vi "Waveform (G3)-Create.vi"(6 "Rep Num":i32, 7 "Name":string, 8 "error in (no error)":errorcluster, 9 "Npts":i32, 10 "Sampling Rate (Hz)":dbl, 11 "Waveform":T1={"Type"=enum."Tone", "Tone"={"Frequency (kHz)"=0.0, "Phase (cycles)"=0.0, "Random phase"=FALSE}, "Pulse Train"={"Pulse width (us)"=0.0, "Pulse rate (Hz)"=0.0, "Gap (ms)"=0.0, "Polarity"=enum."POS", "PT State"={"Template"=[], "Nperiod"=0, "Index"=0, "Pulse Rate (Hz)"=0.0, "Phase (cycles)"=0.0, "Noff"=0}, "Asynch"=FALSE}, "Noise"={"Properties"={"InvFilt"=FALSE, "Aweight"=FALSE, "Seed"=0, "Tokens"=0, "Brickwall"=FALSE}, "Data"={"TokenNum"=0}}, "File"={"Filename"=path "", "Signal"=[], "Channel"=0, "stream"=FALSE, "offset"=0, "nreps"=0, "loops"=0, "Randomize"=FALSE, "order"=[], "Seed"=0, "Tokens"=0}, "FMSweep"={"Rate (oct/s)"=0.0, "Fmin (Hz)"=0.0, "Fmax (Hz)"=0.0, "Ramp (ms)"=0.0, "Linear"=FALSE}, "Chirp Train"={"Params"={"Fmin (kHz)"=4.0, "Fmax (kHz)"=64.0, "Compensate"=FALSE, "Duration (ms)"=2.0}, "Data"={"WF"=[]}}, "Complex Tone"={"Params"={"F0 (Hz)"=0.0, "Band"={"Flow (Hz)"=0.0, "Fhigh (Hz)"=0.0}, "Phase"=enum."Cosine", "Min F0 (Hz)"=0.0, "Max F0 (Hz)"=0.0, "ContinRandPhase"=FALSE, "Max peak factor"=inf, "Max mod depth"=2.0, "MinHarmNum"=0, "MaxHarmNum"=0, "Level Mode"=enum."per component", "% jitter"=0.0}, "Data"={"Ncomp"=0, "MinHarm"=0, "Phase"=[], "Amplitude"=[], "Npts/frame"=0, "Last F0"=0.0, "Fmin"=0.0, "Fmax"=0.0, "Lslope"=0.0, "randphase"=FALSE, "overall rms"=FALSE, "fmult"=[], "jittered"=FALSE}}, "FM"={"Carrier (kHz)"=0.0, "ModRate (Hz)"=0.0, "Depth (Hz)"=0.0, "Phase (cycles)"=0.0}, "Vowel"={"Freqs"="", "Set level"=enum."Total", "Freq"=[], "weights"=[]}, "Ramp"={"Duration (ms)"=0.0}}) -> (0 "error out":errorcluster, 2 "Signal":dbl[](array[numeric]), 3 "Waveform out":T1={"Type"=enum."Tone", "Tone"={"Frequency (kHz)"=0.0, "Phase (cycles)"=0.0, "Random phase"=FALSE}, "Pulse Train"={"Pulse width (us)"=0.0, "Pulse rate (Hz)"=0.0, "Gap (ms)"=0.0, "Polarity"=enum."POS", "PT State"={"Template"=[], "Nperiod"=0, "Index"=0, "Pulse Rate (Hz)"=0.0, "Phase (cycles)"=0.0, "Noff"=0}, "Asynch"=FALSE}, "Noise"={"Properties"={"InvFilt"=FALSE, "Aweight"=FALSE, "Seed"=0, "Tokens"=0, "Brickwall"=FALSE}, "Data"={"TokenNum"=0}}, "File"={"Filename"=path "", "Signal"=[], "Channel"=0, "stream"=FALSE, "offset"=0, "nreps"=0, "loops"=0, "Randomize"=FALSE, "order"=[], "Seed"=0, "Tokens"=0}, "FMSweep"={"Rate (oct/s)"=0.0, "Fmin (Hz)"=0.0, "Fmax (Hz)"=0.0, "Ramp (ms)"=0.0, "Linear"=FALSE}, "Chirp Train"={"Params"={"Fmin (kHz)"=4.0, "Fmax (kHz)"=64.0, "Compensate"=FALSE, "Duration (ms)"=2.0}, "Data"={"WF"=[]}}, "Complex Tone"={"Params"={"F0 (Hz)"=0.0, "Band"={"Flow (Hz)"=0.0, "Fhigh (Hz)"=0.0}, "Phase"=enum."Cosine", "Min F0 (Hz)"=0.0, "Max F0 (Hz)"=0.0, "ContinRandPhase"=FALSE, "Max peak factor"=inf, "Max mod depth"=2.0, "MinHarmNum"=0, "MaxHarmNum"=0, "Level Mode"=enum."per component", "% jitter"=0.0}, "Data"={"Ncomp"=0, "MinHarm"=0, "Phase"=[], "Amplitude"=[], "Npts/frame"=0, "Last F0"=0.0, "Fmin"=0.0, "Fmax"=0.0, "Lslope"=0.0, "randphase"=FALSE, "overall rms"=FALSE, "fmult"=[], "jittered"=FALSE}}, "FM"={"Carrier (kHz)"=0.0, "ModRate (Hz)"=0.0, "Depth (Hz)"=0.0, "Phase (cycles)"=0.0}, "Vowel"={"Freqs"="", "Set level"=enum."Total", "Freq"=[], "weights"=[]}, "Ramp"={"Duration (ms)"=0.0}})   [LabVIEW 2020]
doc: "Takes a generic waveform description and returns a token of the specific waveform."
uses:
  XControls/Waveform XControls/Waveform (G3)/Waveform Data.ctl
  Waveform Enum (V3).ctl
  XControls/Waveform XControls/Tone (G3)/Tone.Properties.ctl
  Waveform VIs/Pulse Train VIs/Pulse Train Params.ctl
  Waveform VIs/Pulse Train VIs/Pulse Polarity.ctl
  Waveform VIs/Pulse Train VIs/PT-Continuous State.ctl
  Noise VIs/Noise (G3).ctl
  Noise VIs/Noise (G3).Properties.ctl
  Noise VIs/Noise (G3).Data.ctl
  Waveform VIs/File VIs/StimFile-Params.ctl
  Waveform VIs/FM Sweep VIs/FM Sweep Params.ctl
  Waveform VIs/Chirp Train VIs/Chirp Train.ctl
  Waveform VIs/Chirp Train VIs/Chirp Train Params.ctl
  Waveform VIs/Complex Tone VIs/CT-Params.ctl
  Waveform VIs/Complex Tone VIs/CT-Phase Enum.ctl
  Waveform VIs/Complex Tone VIs/CT-Runtime Data.ctl
  XControls/Waveform XControls/FM Tone/Data.ctl
  XControls/Waveform XControls/Vowel/Vowel.Properties.ctl
  Ramp VIs/Ramp.Properties.ctl
  XControls/Waveform XControls/Waveform (G3)/Waveform (G3).xctl
  XControls/Waveform XControls/Tone (G3)/Tone (G3).xctl
  XControls/Waveform XControls/FM Tone/FM Tone.xctl
  XControls/Waveform XControls/Vowel/Vowel.xctl
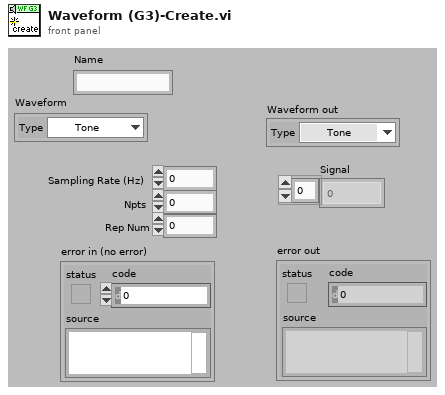
[diagram p1: front panel]
types:
  T1 = typedef "Waveform (G3).xctl/Waveform Data.ctl" = cluster{"Type":T2, "Tone":T3, "Pulse Train":T4, "Noise":T7, "File":T10, "FMSweep":T11, "Chirp Train":T12, "Complex Tone":cluster{"Params":T14, "Data":T16}, "FM":T17, "Vowel":T18, "Ramp":T19}
  T2 = typedef "Waveform Enum (V3).ctl" = enum16{"OFF", "Tone", "Noise", "Pulse Train", "File", "FM Sweep", "Chirp Train", "Complex Tone", "FM Tone", "Vowel", "Ramp"}
  T3 = typedef "Tone (G3).xctl/Tone.Properties.ctl" = cluster{"Frequency (kHz)":dbl, "Phase (cycles)":dbl, "Random phase":bool}
  T4 = typedef "Pulse Train Params.ctl" = cluster{"Pulse width (us)":dbl, "Pulse rate (Hz)":dbl, "Gap (ms)":dbl, "Polarity":T5, "PT State":T6, "Asynch":bool}
  T5 = typedef "Pulse Polarity.ctl" = enum16{"POS", "NEG", "POS-NEG", "NEG-POS"}
  T6 = typedef "PT-Continuous State.ctl" = cluster{"Template":dbl[], "Nperiod":i32, "Index":i32, "Pulse Rate (Hz)":dbl, "Phase (cycles)":dbl, "Noff":i32}
  T7 = typedef "Noise (G3).ctl" = cluster{"Properties":T8, "Data":T9}
  T8 = typedef "Noise (G3).Properties.ctl" = cluster{"InvFilt":bool, "Aweight":bool, "Seed":i32, "Tokens":i32, "Brickwall":bool}
  T9 = typedef "Noise (G3).Data.ctl" = cluster{"TokenNum":i32}
  T10 = typedef "StimFile-Params.ctl" = cluster{"Filename":path, "Signal":dbl[], "Channel":i32, "stream":bool, "offset":i32, "nreps":i32, "loops":i32, "Randomize":bool, "order":i32[], "Seed":i32, "Tokens":i32}
  T11 = typedef "FM Sweep Params.ctl" = cluster{"Rate (oct/s)":dbl, "Fmin (Hz)":dbl, "Fmax (Hz)":dbl, "Ramp (ms)":dbl, "Linear":bool}
  T12 = typedef "Chirp Train.ctl" = cluster{"Params":T13, "Data":cluster{"WF":dbl[]}}
  T13 = typedef "Chirp Train Params.ctl" = cluster{"Fmin (kHz)":dbl, "Fmax (kHz)":dbl, "Compensate":bool, "Duration (ms)":dbl}
  T14 = typedef "CT-Params.ctl" = cluster{"F0 (Hz)":dbl, "Band":cluster{"Flow (Hz)":dbl, "Fhigh (Hz)":dbl}, "Phase":T15, "Min F0 (Hz)":dbl, "Max F0 (Hz)":dbl, "ContinRandPhase":bool, "Max peak factor":dbl, "Max mod depth":dbl, "MinHarmNum":i32, "MaxHarmNum":i32, "Level Mode":enum16{"per component", "overall rms"}, "% jitter":dbl}
  T15 = typedef "CT-Phase Enum.ctl" = enum16{"Cosine", "Random", "Alternating"}
  T16 = typedef "CT-Runtime Data.ctl" = cluster{"Ncomp":i32, "MinHarm":i32, "Phase":dbl[], "Amplitude":dbl[], "Npts/frame":i32, "Last F0":dbl, "Fmin":dbl, "Fmax":dbl, "Lslope":dbl, "randphase":bool, "overall rms":bool, "fmult":dbl[], "jittered":bool}
  T17 = typedef "FM Tone.xctl/Data.ctl" = cluster{"Carrier (kHz)":dbl, "ModRate (Hz)":dbl, "Depth (Hz)":dbl, "Phase (cycles)":dbl}
  T18 = typedef "Vowel.xctl/Vowel.Properties.ctl" = cluster{"Freqs":string, "Set level":enum16{"Total", "Per component"}, "Freq":dbl[], "weights":dbl[]}
  T19 = typedef "Ramp.Properties.ctl" = cluster{"Duration (ms)":dbl}
  T20 = typedef "Tone.Properties.ctl" = cluster{"Frequency (kHz)":dbl, "Phase (cycles)":dbl, "Random phase":bool}
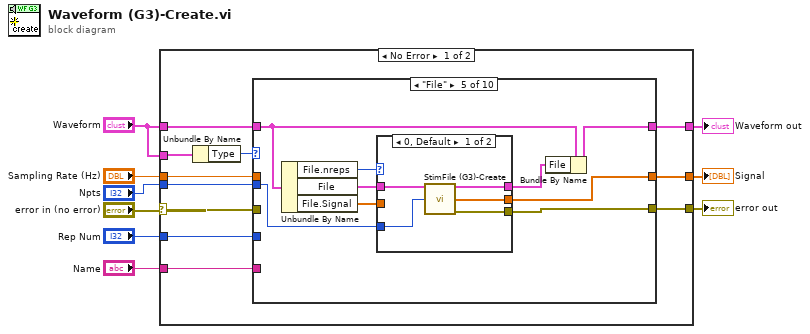
[diagram p0: block diagram]
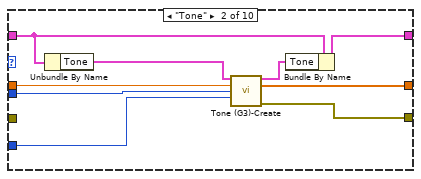
[diagram p3: hidden frame]
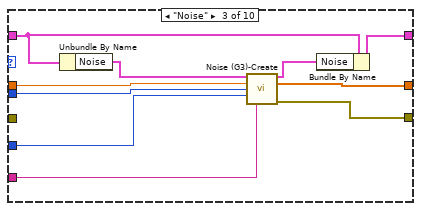
[diagram p4: hidden frame]
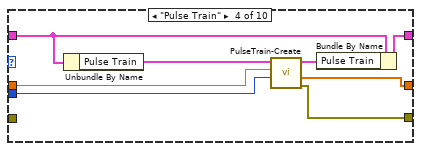
[diagram p5: hidden frame]
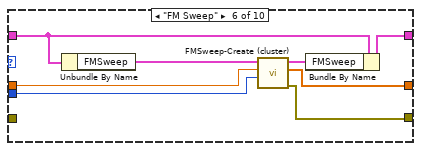
[diagram p7: hidden frame]
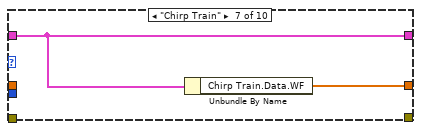
[diagram p8: hidden frame]
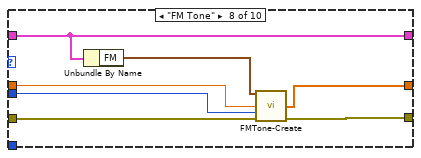
[diagram p9: hidden frame]
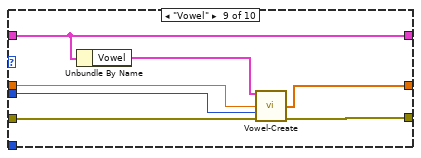
[diagram p10: hidden frame]
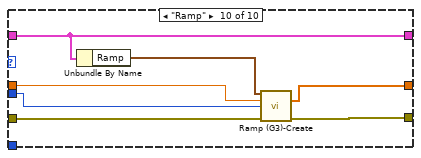
[diagram p11: hidden frame]
diagram:
  n1 = case shown="No Error" "error in (no error)" {
    selector: "error in (no error)" -> [w10 w97]
    tunnel: [w15 w97] -> w8
    tunnel: "Waveform" -> [w20 _]
    tunnel: "Sampling Rate (Hz)" -> [w18 _]
    tunnel: "Npts" -> [w17 _]
    tunnel: "Waveform" -> [w16 w96]
    tunnel: [w14 _] -> w4
    tunnel: [w13 w96] -> w3
    tunnel: "Name" -> [w12 _]
    tunnel: "Rep Num" -> [w11 _]
    frame No Error {
      n2 = Unbundle By Name(w20) -> ("Type"=w19:T2)
      n3 = case shown="\"File\"" w19 {
        tunnel: w18 -> [_ w30 w40 w46 _ w66 _ w76 w83 w91]
        tunnel: w17 -> [_ w29 w39 w45 w52 w65 _ w75 w82 w90]
        tunnel: w16 -> [w21 w28 w38 w48 w57 w72 w74 w81 w88 w95]
        tunnel: [_ w27 w36 w44 w50 w68 _ w79 w86 w93] -> w15
        tunnel: [_ w26 w35 w43 w51 w67 w73 w78 w85 w92] -> w14
        tunnel: [w21 w25 w34 w42 w56 w70 w74 w81 w88 w95] -> w13
        tunnel: w12 -> [_ _ w33 _ _ _ _ _ _ _]
        tunnel: w11 -> [_ w22 w31 _ _ _ _ _ _ _]
        tunnel: w10 -> [_ _ _ _ _ _ _ w80 w87 w94]
        frame "OFF", Default {
        }
        frame "Tone" {
          n4 = Unbundle By Name(w28) -> ("Tone"=w24:T3)
          n5 = call "Tone (G3)-Create.vi"("Tone Class in"=w24, "Sampling Rate (Hz)"=w30, "Npts"=w29, "RepNum"=w22) -> ("Tone Class out"=w23:T20, "Waveform"=w26:dbl[], "error out"=w27:errorcluster)  [unwired: 9 in]
          n6 = Bundle By Name(cluster=w28, "Tone"=w23) -> (w25:T1)
        }
        frame "Noise" {
          n7 = Unbundle By Name(w38) -> ("Noise"=w32:T7)
          n8 = call "Noise (G3)-Create.vi"("Noise In"=w32, "Sampling Rate (Hz)"=w40, "Npts"=w39, "Rep"=w31, "Name"=w33) -> ("Noise Out"=w37:T7, "Waveform"=w35:dbl[], "error out"=w36:errorcluster)  [unwired: 8 in]
          n9 = Bundle By Name(cluster=w38, "Noise"=w37) -> (w34:T1)
        }
        frame "Pulse Train" {
          n10 = Unbundle By Name(w48) -> ("Pulse Train"=w47:T4)
          n11 = call "PulseTrain-Create.vi"("Npts"=w45, "Sampling Rate (Hz)"=w46, "Pulse Train Params"=w47) -> ("error out"=w44:errorcluster, "Waveform"=w43:dbl[], "Pulse Train Params (out)"=w41:T4)  [unwired: 5 in, 1 out]
          n12 = Bundle By Name(cluster=w48, "Pulse Train"=w41) -> (w42:T1)
        }
        frame "File" {
          n13 = Unbundle By Name(w57) -> ("File.nreps"=w55:i32, "File"=w54:T10, "File.Signal"=w53:dbl[])
          n14 = case shown="0, Default" w55 {
            tunnel: w54 -> [w62 w64]
            tunnel: [w61 w64] -> w49
            tunnel: [w60 w63] -> w51
            tunnel: w53 -> [_ w63]
            tunnel: w52 -> [w58 _]
            tunnel: [w59 _] -> w50
            frame 0, Default {
              n15 = call "StimFile (G3)-Create.vi"("File"=w62, "Npts"=w58) -> ("File out"=w61:T10, "Y"=w60:dbl[], "error out"=w59:errorcluster)  [unwired: 11 in]
            }
            frame 1 {
            }
          }
          n16 = Bundle By Name(cluster=w57, "File"=w49) -> (w56:T1)
        }
        frame "FM Sweep" {
          n17 = Unbundle By Name(w72) -> ("FMSweep"=w71:T11)
          n18 = call "FMSweep-Create (cluster).vi"("Npts"=w65, "Sampling Rate (Hz)"=w66, "FMSweep In"=w71) -> ("error out"=w68:errorcluster, "Waveform"=w67:dbl[], "FMSweep Out"=w69:T11)  [unwired: 6 in]
          n19 = Bundle By Name(cluster=w72, "FMSweep"=w69) -> (w70:T1)
        }
        frame "Chirp Train" {
          n20 = Unbundle By Name(w74) -> ("Chirp Train.Data.WF"=w73:dbl[])
        }
        frame "FM Tone" {
          n21 = Unbundle By Name(w81) -> ("FM"=w77:T17)
          n22 = call "FMTone-Create.vi"("FM"=w77, "Sampling Rate (Hz)"=w76, "Npts"=w75, "error in (no error)"=w80) -> ("WF"=w78:dbl[], "error out"=w79:errorcluster)  [unwired: 10 in]
        }
        frame "Vowel" {
          n23 = Unbundle By Name(w88) -> ("Vowel"=w84:T18)
          n24 = call "Vowel-Create.vi"("Vowel"=w84, "Sampling Rate (Hz)"=w83, "Npts"=w82, "error in (no error)"=w87) -> ("WF"=w85:dbl[], "error out"=w86:errorcluster)  [unwired: 10 in]
        }
        frame "Ramp" {
          n25 = Unbundle By Name(w95) -> ("Ramp"=w89:T19)
          n26 = call "Ramp (G3)-Create.vi"("Ramp in"=w89, "Sampling Rate (Hz)"=w91, "Npts"=w90, "error in (no error)"=w94) -> ("Waveform"=w92:dbl[], "error out"=w93:errorcluster)  [unwired: 9 in, 1 out]
        }
      }
    }
    frame Error {
    }
  }
  "error out" <- w8
  "Signal" <- w4
  "Waveform out" <- w3
